vi "Intan_mainControlPanel.vi"() -> ()   [LabVIEW 2015]
panel:
  out "Serial Port Type":string
  out "DT samp (us)":dbl
  out "ADC calib":bool
  in  "Config Hardware Filter":bool=TRUE
  in  "Start Data Stream":bool
  out "HeaderFilePath":path
  in  "Save Display Data":bool
  in  "ConfigReg [0:7, aPwr]":bool=TRUE
  out "Config Result":string
  out "Teensy response":string
  out "actual fs (Hz)":dbl
  out "Raw data file path":path
  in  "Save Raw Data":bool=TRUE
  in  "Desired Fs (Hz)":u16=200
  in  "VISA resource name":refnum<visa-resource-name>="COM33"
  in  "R_L source":u8(ring)=1 items=["ON-chip", "OFF-chip"]
  in  "Lower cutoff":u8(ring)=12 items=["10 Hz", "7.5 Hz", "5.0 Hz", "3.0 Hz", "2.5 Hz", "2.0 Hz", "1.5 Hz", "1.0 Hz", "0.75 Hz", "0.5 Hz", "0.3 Hz", "0.25 Hz", "0.10 Hz"]
  in  "Upper cutoff":u8(ring)=12 items=["5.0 kHz", "3.0 kHz", "2.5 kHz", "2.0 kHz", "1.5 kHz", "1.0 kHz", "750 Hz", "500 Hz", "300 Hz", "250 Hz", "200 Hz", "150 Hz", "100 Hz"]
  # "Intan-Teensy Bioelectric Module: configure hardware and serial port (32ch)"
  # "Configure all settings, then click run arrow.\n\nWhen config is complete, click the purple\nbutton to start data stream.\n\nSeparate VI will pop open to display signals"
  # "TODO 01 May 2017 JE\n\nSTATUS: Operational, beta.\n\nSOFTWARE issues:\n\n - Set decimation ratio to ensure Nsamps in display never exceeds chart limit\nor sensible human visibility bound (for now set chart history length = 50000.\nFor typical max sampling rates of 500 Hz in our applications, this still allows up to 100 s\nof data display (ridiculously long).  In practice, could probably increase performance\nby decreasing chart history to something smaller like 20000.\n\n\n- Make bdf style header and write to file (low priority)\n\n -  Stream to main fig window, Present only does this in subVI (IntanStream_Parallel Loops.vi)\n  SOLN: just pop open subVI automatically when called, but pre-set filters (?)\n\nHARDWARE issues: \n\n\nNeed to gracefully recover when data sync is lost. Option to reboot Teensy and recover connection? \nCurrent error checking not working, don' know why.  Software reset tricky to implement:\nhttps://forum.pjrc.com/archive/index.php/t-24304.html\nBest solution for now, unplug then replug power.  This puts Teensy back into initial state.\n\n-Option to stream subset of channels.  This will allow higher data rate for wireless streaming, if desired."
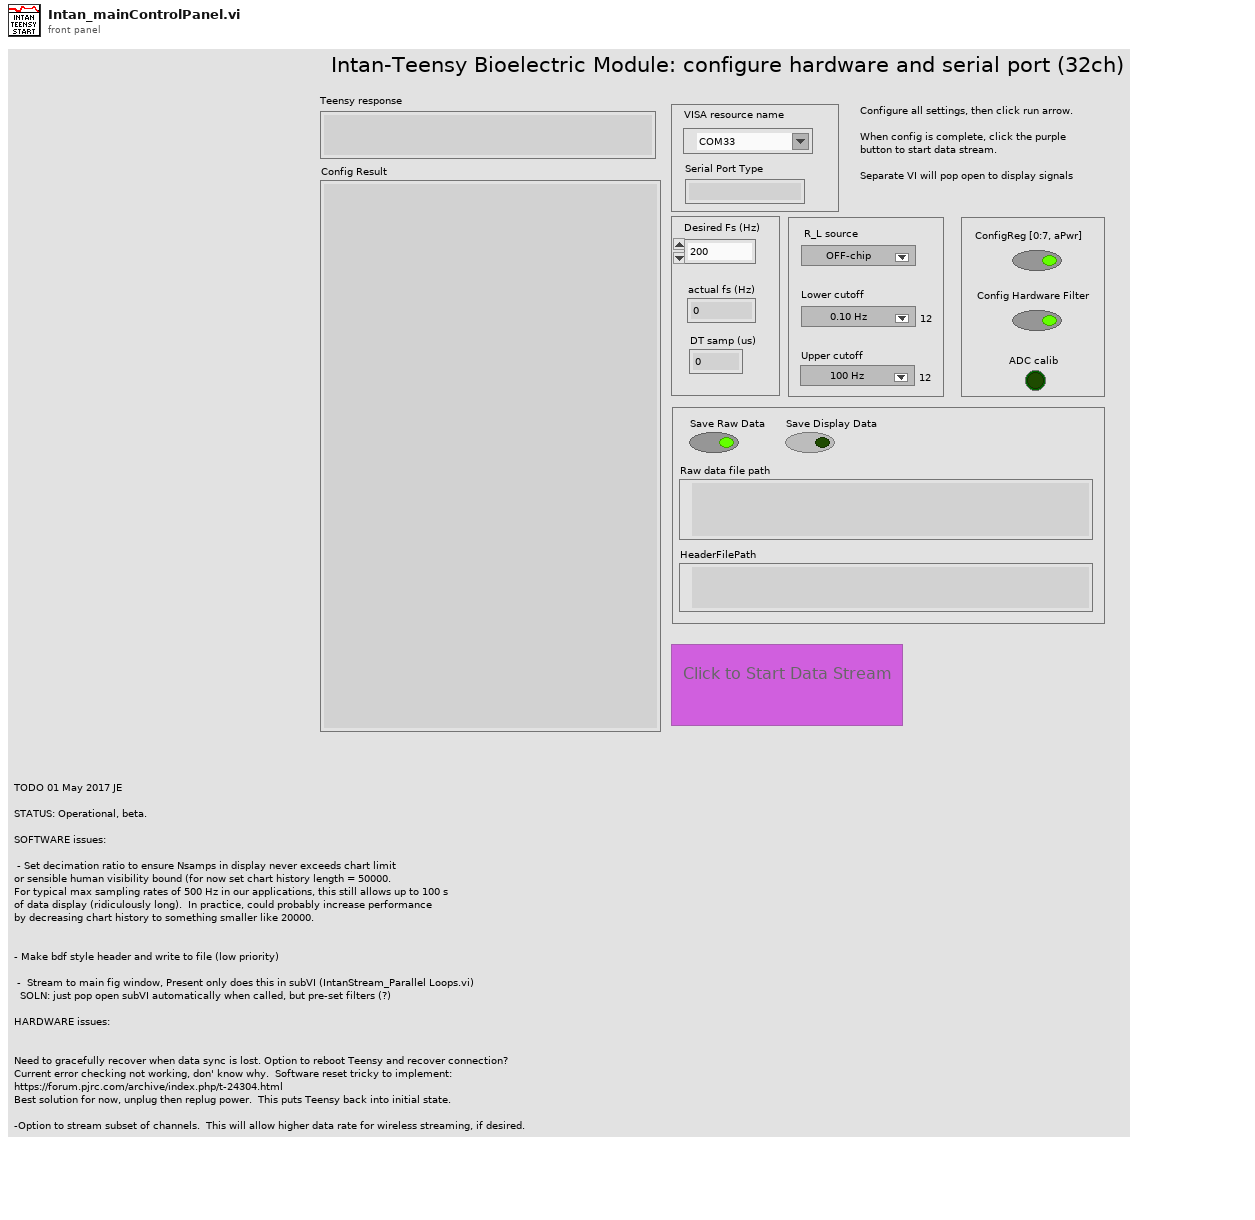
[diagram p1: front panel]
types:
  T1 = enum8{"Enabled", "Disabled", "Disabled and Grayed Out"}
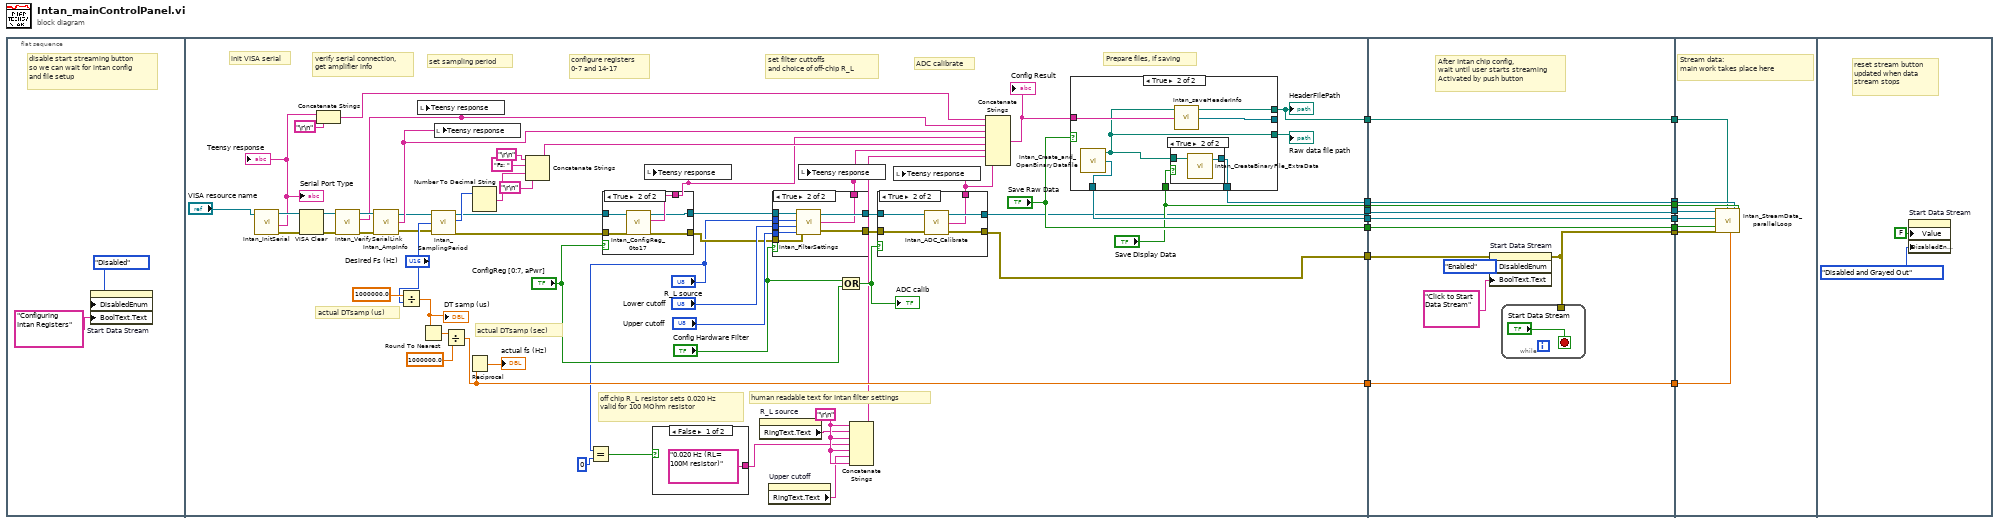
[diagram p0: block diagram]
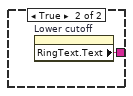
[diagram p2: hidden frame]
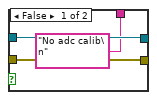
[diagram p3: hidden frame]
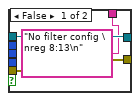
[diagram p4: hidden frame]
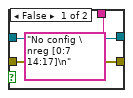
[diagram p5: hidden frame]
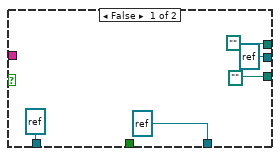
[diagram p6: hidden frame]
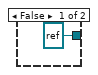
[diagram p7: hidden frame]
diagram:
  n1 = flat-sequence {
    tunnel: [w71] -> w10
    tunnel: [w57] -> w9
    tunnel: [w54] -> w8
    tunnel: ["Save Raw Data"] -> w7
    tunnel: ["Save Display Data"] -> w6
    tunnel: [w40] -> w5
    tunnel: [w39] -> w3
    tunnel: [w33] -> w1
    tunnel: [w125] -> w16
    tunnel: [w131] -> w15
    tunnel: [w130] -> w14
    tunnel: [w129] -> w13
    tunnel: [w128] -> w12
    tunnel: [w127] -> w11
    tunnel: w6 -> [w127]
    tunnel: w7 -> [w128]
    tunnel: w8 -> [w129]
    tunnel: w9 -> [w130]
    tunnel: w10 -> [w131]
    tunnel: w5 -> [w124]
    tunnel: [w123] -> w4
    tunnel: w3 -> [w123]
    tunnel: [w122] -> w2
    tunnel: w1 -> [w122]
    tunnel: w16 -> [w137]
    tunnel: w15 -> [w135]
    tunnel: w14 -> [w140]
    tunnel: w13 -> [w138]
    tunnel: w12 -> [w136]
    tunnel: w11 -> [w139]
    tunnel: w4 -> [w134]
    tunnel: w2 -> [w133]
    frame #0 {
      # "disable start streaming button\nso we can wait for intan config\nand file setup"
      n2 = property on="Start Data Stream" class="Bool (strict)"("DisabledEnum"=T1."Disabled" ("Disabled"), "BoolText.Text"="Configuring Intan Registers" ("Boolean Text.Text")) -> ()  [unwired: 2 in, 2 out]
    }
    frame #1 {
      w27 = "\r\n"
      # "off chip R_L resistor sets 0.020 Hz \nvalid for 100 MOhm resistor"
      # "human readable text for Intan filter settings"
      # "Prepare files, if saving"
      # "ADC calibrate"
      # "set filter cuttoffs \nand choice of off-chip R_L"
      # "configure registers\n0-7 and 14-17"
      # "set sampling period"
      # "verify serial connection,\nget amplifier info"
      # "init VISA serial"
      # "actual DTsamp (sec)"
      # "actual DTsamp (us)"
      n3 = call "Intan_InitSerial.vi"("VISA resource name"="VISA resource name") -> ("VISA resource name out"=w32:refnum<visa-resource-name>, "Text response"=w29:string, "error out"=w69:errorcluster)  [unwired: 3 in]
      "Teensy response" <- w29
      "Serial Port Type" <- w29
      n4 = VISA Clear(VISA resource name=w32, error in (no error)=w69) -> (VISA resource name out=w70:refnum<visa-resource-name>, error out=w68:errorcluster)
      n5 = Concatenate Strings(w29, "\r\n") -> (w30:string)
      n6 = call "Intan_VerifySerialLink.vi"("error in"=w68, "VISA resource name"=w70) -> ("error out"=w72:errorcluster, "Text response"=w66:string, "VISA resource name out"=w73:refnum<visa-resource-name>)  [unwired: 7 in]
      n7 = call "Intan_AmpInfo.vi"("error in"=w72, "VISA resource name"=w73) -> ("error out"=w50:errorcluster, "Text response"=w67:string, "VISA resource name out"=w51:refnum<visa-resource-name>)  [unwired: 1 in]
      n8 = Divide(x=1000000.0, y="Desired Fs (Hz)") -> (x/y=w34:dbl)
      "DT samp (us)" <- w34
      n9 = local write "Teensy response"(w66) -> ()
      n10 = Round To Nearest(number=w34) -> (nearest integer value=w59:dbl)
      n11 = call "Intan_SamplingPeriod.vi"("VISA resource name"=w51, "Desired Fs (Hz)"="Desired Fs (Hz)", "error in"=w50) -> ("VISA resource name out"=w49:refnum<visa-resource-name>, "FS actual (Hz)"=w65:i32, "error out"=w48:errorcluster)  [unwired: 1 out]
      n12 = local write "Teensy response"(w67) -> ()
      n13 = Divide(x=w59, y=1000000.0 ("x")) -> (x/y=w57:dbl)
      n14 = Reciprocal(x=w57) -> (1/x=→"actual fs (Hz)":dbl)
      n15 = Number To Decimal String(number=w65) -> (decimal integer string=w64:string)  [unwired: 1 in]
      n16 = Concatenate Strings("\r\n", "Fs: " ("string"), w64, "\r\n") -> (w62:string)
      n17 = Equal?(x="R_L source", y=u8 0) -> (x = y?=w22:bool)
      n18 = case shown="True" "ConfigReg [0:7, aPwr]" {
        tunnel: w49 -> [w99 w105]
        tunnel: w48 -> [w98 w104]
        tunnel: ["No config \nreg [0:7 14:17]\n" ("Text response") w103] -> w47
        tunnel: [w99 w102] -> w44
        tunnel: [w98 w101] -> w43
        frame False {
        }
        frame True {
          n19 = call "Intan_ConfigReg_0to17.vi"("error in"=w104, "VISA resource name"=w105) -> ("error out"=w101:errorcluster, "Text response"=w103:string, "VISA resource name out"=w102:refnum<visa-resource-name>)  [unwired: 7 in]
        }
      }
      n20 = local write "Teensy response"(w47) -> ()
      n21 = case shown="False" w22 {
        tunnel: ["0.020 Hz (RL= 100M resistor)" ("string") w78] -> w20
        frame False {
        }
        frame True {
          n22 = property on="Lower cutoff" class="Ring (strict)"() -> ("RingText.Text"=w78:string)  [unwired: 2 in, 2 out]
        }
      }
      n23 = property on="R_L source" class="Ring (strict)"() -> ("RingText.Text"=w25:string)  [unwired: 2 in, 2 out]
      n24 = property on="Upper cutoff" class="Ring (strict)"() -> ("RingText.Text"=w26:string)  [unwired: 2 in, 2 out]
      n25 = case shown="True" "Config Hardware Filter" {
        tunnel: "R_L source" -> [_ w97]
        tunnel: "Lower cutoff" -> [_ w96]
        tunnel: "Upper cutoff" -> [_ w95]
        tunnel: w44 -> [w89 w94]
        tunnel: w43 -> [w88 w93]
        tunnel: [w89 w92] -> w42
        tunnel: [w88 w91] -> w41
        tunnel: ["No filter config \nreg 8:13\n" ("Text response") w90] -> w38
        frame False {
        }
        frame True {
          n26 = call "Intan_FilterSettings.vi"("VISA resource name"=w94, "R_L source"=w97, "Lower cutoff"=w96, "Upper cutoff"=w95, "error in"=w93) -> ("VISA resource name out"=w92:refnum<visa-resource-name>, "Text response"=w90:string, "error out"=w91:errorcluster)
        }
      }
      n27 = local write "Teensy response"(w38) -> ()
      n28 = Or(x="Config Hardware Filter", y="ConfigReg [0:7, aPwr]") -> (x .or. y?=w37:bool)
      "ADC calib" <- w37
      n29 = Concatenate Strings(w27, w25, w27, w20, w27, w26, w27) -> (w23:string)
      n30 = case shown="True" w37 {
        tunnel: w42 -> [w81 w86]
        tunnel: w41 -> [w80 w85]
        tunnel: [w80 w84] -> w40
        tunnel: [w81 w83] -> w39
        tunnel: ["No adc calib\n" ("Text response") w82] -> w24
        frame False {
        }
        frame True {
          n31 = call "Intan_ADC_Calibrate.vi"("error in"=w85, "VISA resource name"=w86) -> ("error out"=w84:errorcluster, "Text response"=w82:string, "VISA resource name out"=w83:refnum<visa-resource-name>)  [unwired: 1 in]
        }
      }
      n32 = local write "Teensy response"(w24) -> ()
      n33 = Concatenate Strings(w30, w66, w67, w47, w62, w38, w23, w24) -> (w55:string)
      "Config Result" <- w55
      n34 = case shown="True" "Save Raw Data" {
        tunnel: [refnum<file> refnum ("refnum out") w117] -> w71
        tunnel: w55 -> [_ w116]
        tunnel: [refnum<file> refnum ("refnum out") w115] -> w54
        tunnel: "Save Display Data" -> [_ w114]
        tunnel: [path "" w113] -> w33
        tunnel: [path "" w112] -> w45
        tunnel: [refnum<file> refnum ("hdr_file_ref_num_out") w111] -> _
        frame False {
        }
        frame True {
          n35 = call "Intan_Create_and_OpenBinaryDatafile.vi"() -> ("file path"=w112:path, "refnum out"=w117:refnum<file>)  [unwired: 2 in, 1 out]
          n36 = case shown="True" w114 {
            tunnel: w112 -> [_ w120]
            tunnel: [refnum<file> refnum ("refnum out") w119] -> w115
            frame False {
            }
            frame True {
              n37 = call "Intan_CreateBinaryFile_ExtraData.vi"("DataFilePath"=w120) -> ("refnum out"=w119:refnum<file>)  [unwired: 3 in, 1 out]
            }
          }
          n38 = call "Intan_saveHeaderInfo.vi"("header text"=w116, "DataFilePath"=w112) -> ("hdr_file_ref_num_out"=w111:refnum<file>, "HeaderFilePath"=w113:path)  [unwired: 1 in, 1 out]
        }
      }
      "HeaderFilePath" <- w33
      "Raw data file path" <- w45
    }
    frame #2 {
      # "After Intan chip config,\nwait until user starts streaming\nActivated by push button"
      n39 = property on="Start Data Stream" class="Bool (strict)"(error in=w124, "DisabledEnum"=T1."Enabled" ("Disabled"), "BoolText.Text"="Click to Start Data Stream" ("Boolean Text.Text")) -> (error out=w125:errorcluster)  [unwired: 1 in, 1 out]
      n40 = while {
        tunnel: w125 -> [_]
        stop <- "Start Data Stream" stop-if-true
      }
    }
    frame #3 {
      # "Stream data: \nmain work takes place here"
      n41 = call "Intan_StreamData_parallelLoop.vi"("VISA resource name"=w134, "refnum in"=w135, "Save Binary Data"=w136, "error in"=w137, "hdr fpath"=w133, "DT_scale (sec)"=w140, "aux file ref num"=w138, "save aux file"=w139) -> ()  [unwired: 8 in, 4 out]
    }
    frame #4 {
      # "reset stream button \nupdated when data\nstream stops"
      n42 = property on="Start Data Stream" class="Bool (strict)"("Value"=FALSE ("Start Data Stream"), "DisabledEnum"=T1."Disabled and Grayed Out" ("Disabled")) -> ()  [unwired: 2 in, 2 out]
    }
  }
